vi "CreateStaveMapFromCalibration.vi"() -> ()   [LabVIEW 2016]
uses:
  Controls/All_Enums/Enum_TypeDef_FidMarkers.ctl
  <vilib>/Utility/file.llb/Write Delimited Spreadsheet (DBL).vi
panel:
  in  "Module fiducial marker":T1
  in  "Tooling Pin Orientation":bool=TRUE
  in  "Stave Orientation":bool=TRUE
  out "StaveOrientationString":string
  out "ToolingPinOrientationString":string
  out "zstop to calibration origin":dbl[](array[numeric]) format="%#_10g"
  out "RelCalibrationPoints":dbl[][](array[numeric])=[[0.0, 0.0, 0.0], [1182.0, 0.0, 0.0]]
  out "ZStopToFirstModuleCorners":dbl[][](array[numeric])=[[-5.712, -115.081], [-9.591, -18.079], [89.691, -111.266], [85.812, -14.264]] format="%#_10g"
  out "Before all shifts":dbl[][](array[numeric])=[[-6.410953088255148, 114.4761813813091, 16.157678], [89.03677648970674, 111.99398106460231, 16.157678], [86.51095308825515, 14.868818618690895, 16.157678], [-8.936776489706752, 17.35101893539769, 16.157678], [91.58904691174487, 114.4761813813091, 16.157678], [187.03677648970677, 111.99398106460231, 16.157678], [184.51095308825515, 14.868818618690895, 16.157678], [89.06322351029326, 17.35101893539769, 16.157678], [189.58904691174487, 114.4761813813091, 16.157678], [285.03677648970677, 111.99398106460231, 16.157678], [282.5109530882552, 14.868818618690895, 16.157678], [187.06322351029326, 17.35101893539769, 16.157678], [287.58904691174484, 114.4761813813091, 16.157678], [383.03677648970677, 111.99398106460231, 16.157678], [380.5109530882552, 14.868818618690895, 16.157678], [285.06322351029326, 17.35101893539769, 16.157678], [385.58904691174484, 114.4761813813091, 16.157678], [481.03677648970677, 111.99398106460231, 16.157678], [478.5109530882552, 14.868818618690895, 16.157678], [383.06322351029326, 17.35101893539769, 16.157678], [483.5890469117448, 114.4761813813091, 16.157678], [579.0367764897067, 111.99398106460231, 16.157678], [576.5109530882551, 14.868818618690895, 16.157678], [481.0632235102932, 17.35101893539769, 16.157678], [581.5890469117448, 114.4761813813091, 16.157678], [677.0367764897067, 111.99398106460231, 16.157678], [674.5109530882551, 14.868818618690895, 16.157678], [579.0632235102933, 17.35101893539769, 16.157678], [679.5890469117448, 114.4761813813091, 16.157678], [775.0367764897067, 111.99398106460231, 16.157678], [772.5109530882551, 14.868818618690895, 16.157678], [677.0632235102933, 17.35101893539769, 16.157678], [777.5890469117448, 114.4761813813091, 16.157678], [873.0367764897067, 111.99398106460231, 16.157678], [870.5109530882551, 14.868818618690895, 16.157678], [775.0632235102933, 17.35101893539769, 16.157678], [875.5890469117448, 114.4761813813091, 16.157678], [971.0367764897067, 111.99398106460231, 16.157678], [968.5109530882551, 14.868818618690895, 16.157678], [873.0632235102933, 17.35101893539769, 16.157678], [973.5890469117448, 114.4761813813091, 16.157678], [1069.0367764897067, 111.99398106460231, 16.157678], [1066.510953088255, 14.868818618690895, 16.157678], [971.0632235102933, 17.35101893539769, 16.157678], [1071.5890469117448, 114.4761813813091, 16.157678], [1167.0367764897067, 111.99398106460231, 16.157678], [1164.510953088255, 14.868818618690895, 16.157678], [1069.0632235102933, 17.35101893539769, 16.157678], [1169.5890469117448, 114.4761813813091, 16.157678], [1265.0367764897067, 111.99398106460231, 16.157678], [1262.510953088255, 14.868818618690895, 16.157678], [1167.0632235102933, 17.35101893539769, 16.157678]]
  out "After Translation":dbl[][](array[numeric])=[[-639.0722496134326, -5.341587943318508, 16.157678], [-543.6216669695231, -2.971635847134557, 16.157678], [-546.033269459689, 94.15642980553571, 16.157678], [-641.4838521035986, 91.78647770935177, 16.157678], [-541.0723173792488, -5.456835916754308, 16.157678], [-445.62173473533926, -3.086883820570357, 16.157678], [-448.0333372255052, 94.04118183209991, 16.157678], [-543.4839198694146, 91.67122973591597, 16.157678], [-443.07238514506497, -5.5720838901901075, 16.157678], [-347.62180250115546, -3.2021317940061564, 16.157678], [-350.0334049913214, 93.92593385866411, 16.157678], [-445.48398763523085, 91.55598176248017, 16.157678], [-345.07245291088117, -5.687331863625907, 16.157678], [-249.62187026697168, -3.317379767441956, 16.157678], [-252.03347275713756, 93.81068588522831, 16.157678], [-347.48405540104704, 91.44073378904437, 16.157678], [-247.0725206766974, -5.802579837061707, 16.157678], [-151.62193803278788, -3.4326277408777557, 16.157678], [-154.03354052295376, 93.69543791179251, 16.157678], [-249.48412316686327, 91.32548581560857, 16.157678], [-149.0725884425136, -5.917827810497506, 16.157678], [-53.622005798604185, -3.5478757143135553, 16.157678], [-56.03360828877012, 93.58018993835671, 16.157678], [-151.48419093267952, 91.21023784217277, 16.157678], [-51.072656208329725, -6.033075783933306, 16.157678], [44.37792643557962, -3.663123687749355, 16.157678], [41.9663239454138, 93.46494196492091, 16.157678], [-53.48425869849566, 91.09498986873697, 16.157678], [46.92727602585408, -6.148323757369106, 16.157678], [142.3778586697634, -3.7783716611851546, 16.157678], [139.9662561795976, 93.34969399148514, 16.157678], [44.515673535688144, 90.97974189530117, 16.157678], [144.92720826003787, -6.263571730804905, 16.157678], [240.37779090394733, -3.893619634620954, 16.157678], [237.9661884137814, 93.23444601804934, 16.157678], [142.51560576987194, 90.86449392186537, 16.157678], [242.92714049422167, -6.378819704240705, 16.157678], [338.37772313813116, -4.008867608056754, 16.157678], [335.9661206479652, 93.11919804461354, 16.157678], [240.51553800405574, 90.74924594842958, 16.157678], [340.9270727284055, -6.4940676776765045, 16.157678], [436.37765537231496, -4.124115581492553, 16.157678], [433.96605288214903, 93.00395007117774, 16.157678], [338.5154702382397, 90.63399797499378, 16.157678], [438.9270049625892, -6.609315651112304, 16.157678], [534.3775876064987, -4.239363554928339, 16.157678], [531.965985116333, 92.88870209774194, 16.157678], [436.5154024724235, 90.51875000155798, 16.157678], [536.9269371967731, -6.724563624548104, 16.157678], [632.3775198406826, -4.3546115283641385, 16.157678], [629.9659173505166, 92.77345412430614, 16.157678], [534.5153347066074, 90.40350202812218, 16.157678]]
  in  "Calibration Directory":path=path "C:/Users/Aerotech/Documents/Zach/Test_5"
  in  "Code path":path=path "C:/Users/Aerotech/Documents/BNL_ThermomechanicalStave"
  # "CREATE STAVE MAP FROM CALIBRATION Brandeis University - Brookhaven National Laboratory * ATLAS Phase II Inner Tracker Upgrade\nPrimary Author: Hannah Herde (hherde@brandeis.edu)"
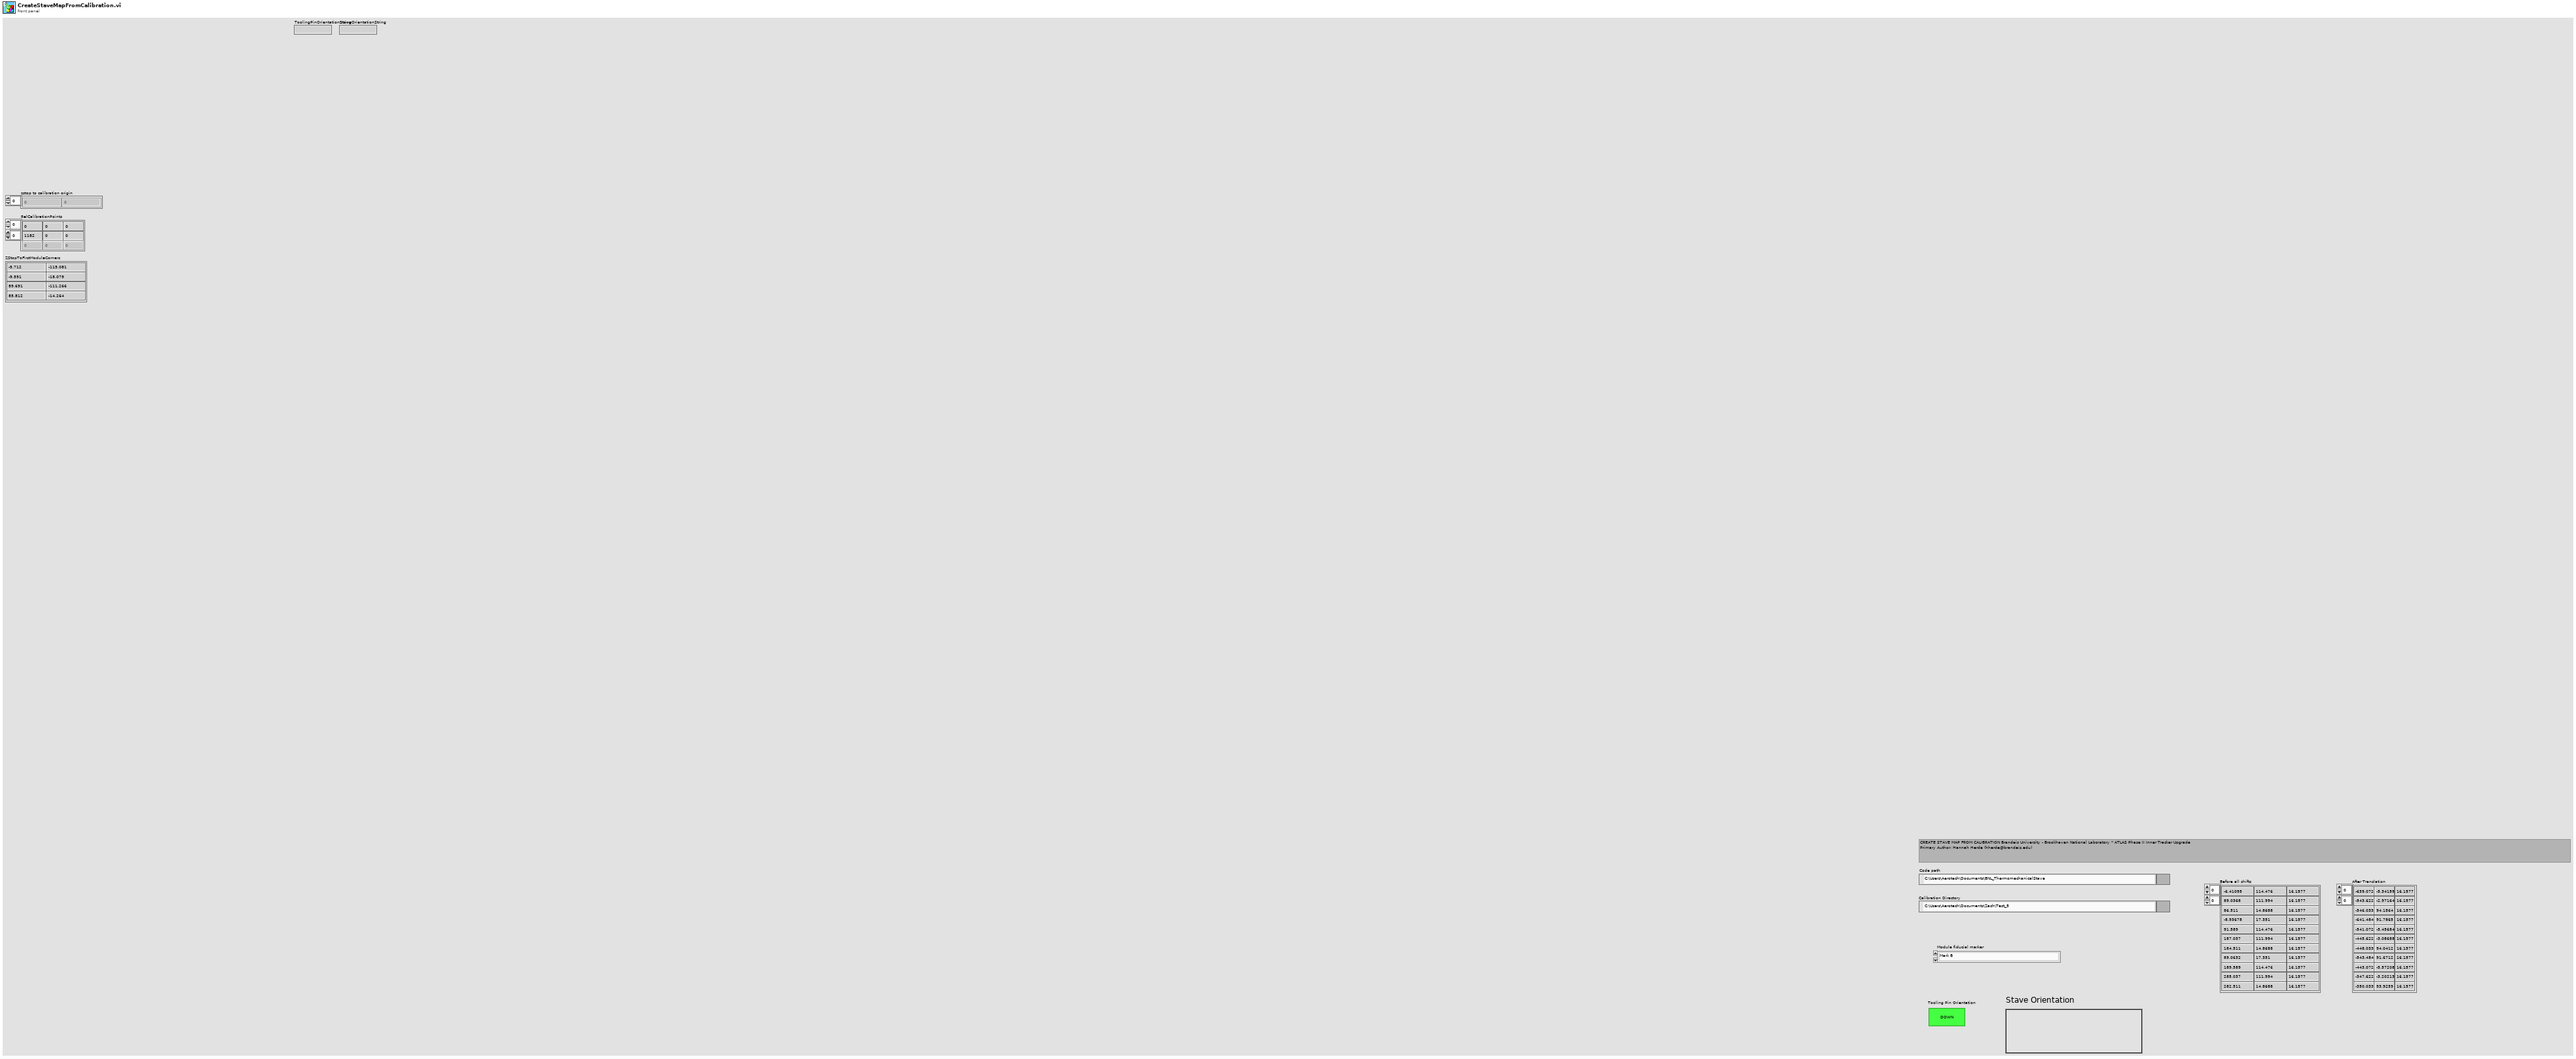
[diagram p1: front panel]
types:
  T1 = typedef "Enum_TypeDef_FidMarkers.ctl" = enum16{"Mark B", "Mark C", "Bias Ring Corner", "Mark I (Slim/17)", "Mark E (Slim/17)", "Mark F (Slim/17)", "Mark G (Slim/17)", "Mark A (12)", "Kapton Spacers"}
  T2 = typedef "Enum_TypeDef_Sensors.ctl" = enum16{"ATLAS07", "ATLAS12", "ATLAS12Slim", "ATLAS17LS"}
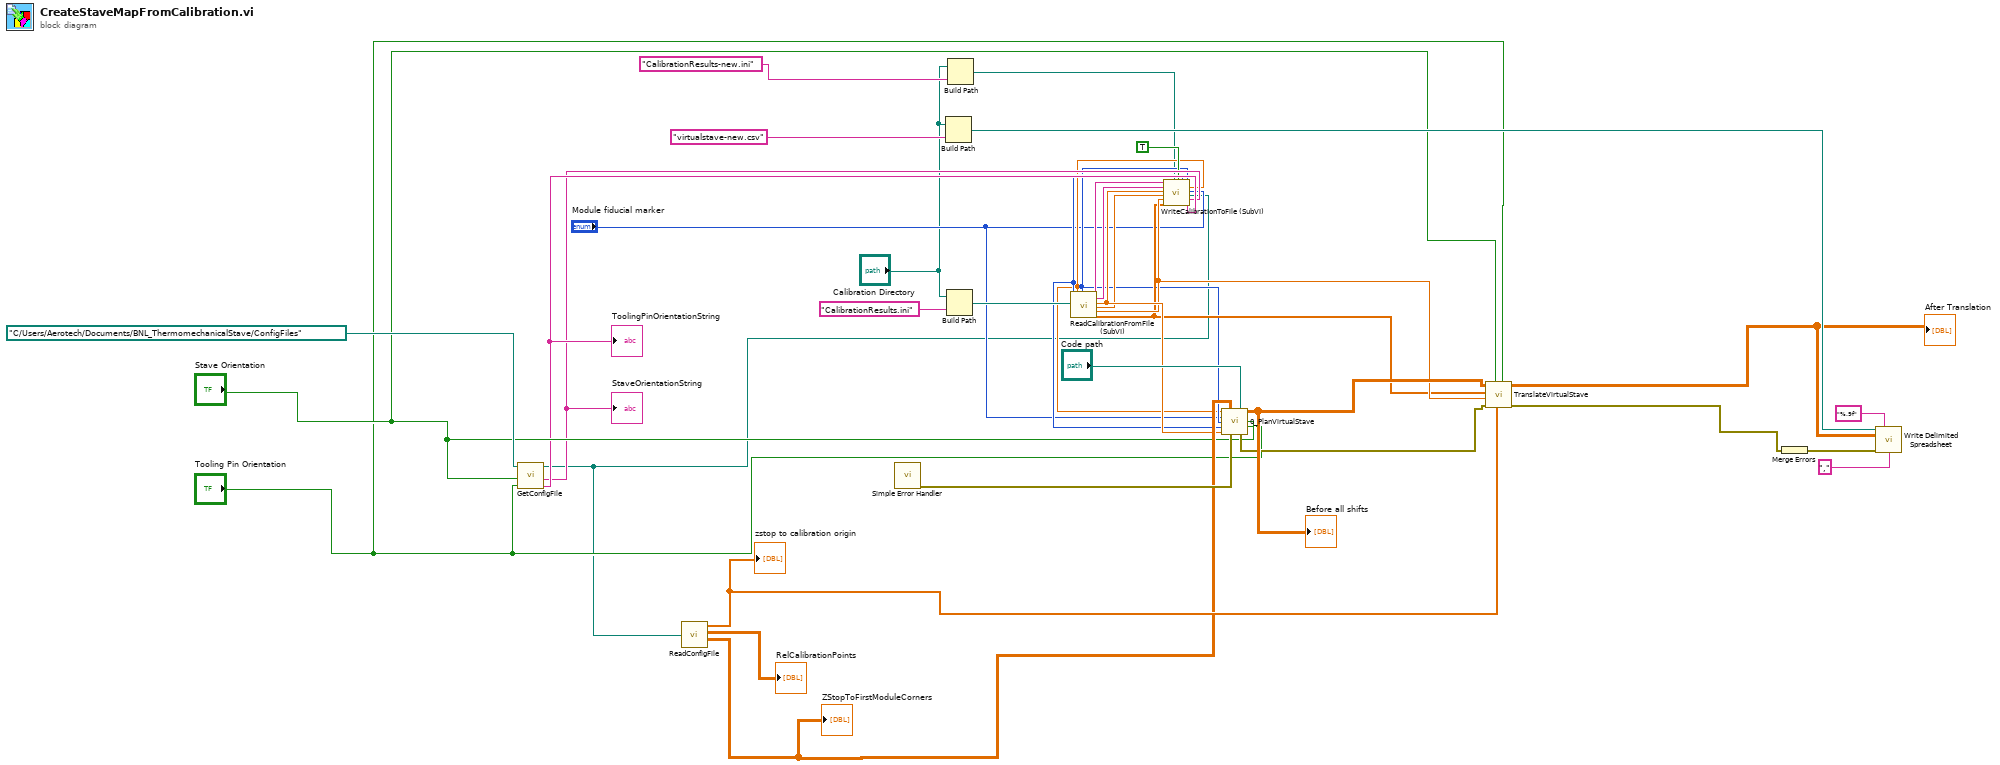
[diagram p0: block diagram]
diagram:
  n1 = call "GetConfigFile.vi"("Tooling Pin Orientation"="Tooling Pin Orientation", "Stave Orientation"="Stave Orientation", "base path"=path "C:/Users/Aerotech/Documents/BNL_ThermomechanicalStave/ConfigFiles") -> ("ToolingPinOrientationString"=w11:string, "StaveOrientationString"=w10:string, "Stave Configuration File"=w4:path)  [unwired: 1 in, 1 out]
  "ToolingPinOrientationString" <- w11
  "StaveOrientationString" <- w10
  n2 = call "ReadConfigFile.vi"("path to config file"=w4) -> ("zstop to calibration origin"=w22:dbl[], "rel. location of calibration points"=→"RelCalibrationPoints":dbl[][], "zstop to first module corners"=w21:dbl[][])  [unwired: 1 out]
  "ZStopToFirstModuleCorners" <- w21
  "zstop to calibration origin" <- w22
  n3 = call <vilib>:"Simple Error Handler.vi"() -> ("error out"=w31:errorcluster)  [unwired: 5 in, 4 out]
  n4 = Build Path(base path="Calibration Directory", name or relative path="virtualstave-new.csv") -> (appended path=w35:path)
  n5 = Build Path(base path="Calibration Directory", name or relative path="CalibrationResults.ini") -> (appended path=w28:path)
  n6 = Build Path(base path="Calibration Directory", name or relative path="CalibrationResults-new.ini") -> (appended path=w1:path)
  n7 = call "ReadCalibrationFromFile (SubVI).vi"("Calibration file path"=w28) -> ("N Modules"=w8:i32, "Stereo angle [mrad]"=w6:dbl, "Sensor pattern"=w7:T2, "Stave ID"=w16:string, "User notes"=w17:string, "CameraWD"=w15:dbl, "um/Pixel"=w14:dbl, "Angle"=w13:dbl, "Stave Origin"=w12:dbl[])  [unwired: 7 in, 3 out]
  n8 = call "WriteCalibrationToFile (SubVI).vi"("Stave ID"=w16, "User notes"=w17, "CameraWD"=w15, "um/Pixel"=w14, "Angle"=w13, "Stave Origin"=w12, "Calibration file path"=w1, "Write to file"=TRUE, "N Modules"=w8, "Sensor pattern"=w7, "Stereo angle [mrad]"=w6, "Module fiducial marker"="Module fiducial marker", "Stave Configuration File"=w4, "StaveOrientationString"=w10, "ToolingPinOrientationString"=w11) -> ()  [unwired: 4 in, 1 out]
  n9 = call "0_PlanVirtualStave.vi"("Stereo Angle [mrad]"=w6, "ZStopToFirstModuleCorners"=w21, "Code path"="Code path", "Module fiducial marker"="Module fiducial marker", "Sensor Pattern"=w7, "Stave Orientation"="Stave Orientation", "N Modules"=w8, "Tooling Pin Orientation"="Tooling Pin Orientation", "Working height [mm]"=w15, "error in (no error)"=w31) -> ("Stave Basis: Coordinates of Fiducials on Modules"=w26:dbl[][], "error out"=w25:errorcluster)  [unwired: 3 in, 1 out]
  "Before all shifts" <- w26
  n10 = call "TranslateVirtualStave.vi"("Tooling Pin Orientation"="Tooling Pin Orientation", "ZStopToCalibrationOrigin"=w22, "Stave Orientation"="Stave Orientation", "error in"=w25, "Angle between stave and xyz stage"=w13, "Calibrated stave origin (X,Y) [mm]"=w12, "Stave Basis: Coordinates of Fiducials on Modules"=w26) -> ("Error out"=w24:errorcluster[], "Virtual Stave"=w23:dbl[][])  [unwired: 3 in]
  "After Translation" <- w23
  n11 = Merge Errors(w24) -> (w33:errorcluster)
  n12 = call-poly <vilib>:"Write Delimited Spreadsheet.vi"("file path (dialog if empty)"=w35, "format (%.3f)"="%.9f", "2D data"=w23, "error in (no error)"=w33, "delimiter (\\t)"="," ("delimiter (\\t)")) -> ()  [unwired: 9 in, 2 out]
